vi "Tosca-Execute Flowchart.vi"(0 "Tosca":refnum<class "Parameters.lvclass">, 1 "StimCon":T1, 2 "IPC":T7, 7 "AODO":T4[](array[typedef]), 11 "error in":errorcluster, 13 "Control Refs":T9) -> (4 "Result":T8, 6 "History":string[](array[string]), 8 "Result string":string, 10 "Rxn time":i32, 14 "Abort":bool, 15 "error out":errorcluster)   [LabVIEW 2020]
uses:
  Typedefs/Tosca-Control Refs.ctl
  FSM Graph VIs/LV Source/FSM Editor/FSM Editor.xctl
  Typedefs/Tosca-Trial Result Enum.ctl
  IPC VIs/Tosca-IPC.ctl
  Classes/Parameters/Parameters.lvclass
  Digital Input VIs/Tosca-DI Queue Data.ctl
  Digital Input VIs/Tosca-Input Event.ctl
  Digital Input VIs/Tosca-Input Criterion.ctl
  epl-vi-lib/Utility VIs/Type Defs/Logic State.ctl
  Typedefs/Tosca-Accumulator.ctl
  Typedefs/Tosca-State AODO.ctl
  Typedefs/Tosca-AO Runtime.ctl
  Typedefs/Tosca-DO Runtime.ctl
  epl-vi-lib/Signal Synthesis VIs/4th Generation/Classes/SignalManager/SignalManager.lvclass
  Typedefs/Tosca-Synapse Start Data.ctl
  IPC VIs/Tosca-Message.ctl
  IPC VIs/Tosca-Message Action.ctl
  Typedefs/Tosca-Thread Type.ctl
  Imaging VIs/Tosca-2P-Notifier Data.ctl
  Typedefs/Tosca-MATLAB Queue Data.ctl
  Visual Stim VIs/Tosca-Grating.ctl
  Visual Stim VIs/Tosca-Grating Type.ctl
  Typedefs/Tosca-File IO Notification.ctl
  Typedefs/Tosca-SCL Element.ctl
  Typedefs/Tosca-Schedule Mode.ctl
  Typedefs/Tosca-Event Type.ctl
  Trace VIs/Tosca-Trace-Event.ctl
  Classes/Parameters/Parameters.lvclass/Parameters.ctl
  Classes/Parameters/Read Flowchart.vi
  Classes/Parameters/Read First state.vi
  Classes/Parameters/Read Target state.vi
  Classes/State/State.lvclass
panel:
  out "Tosca out":refnum<class "Parameters.lvclass">
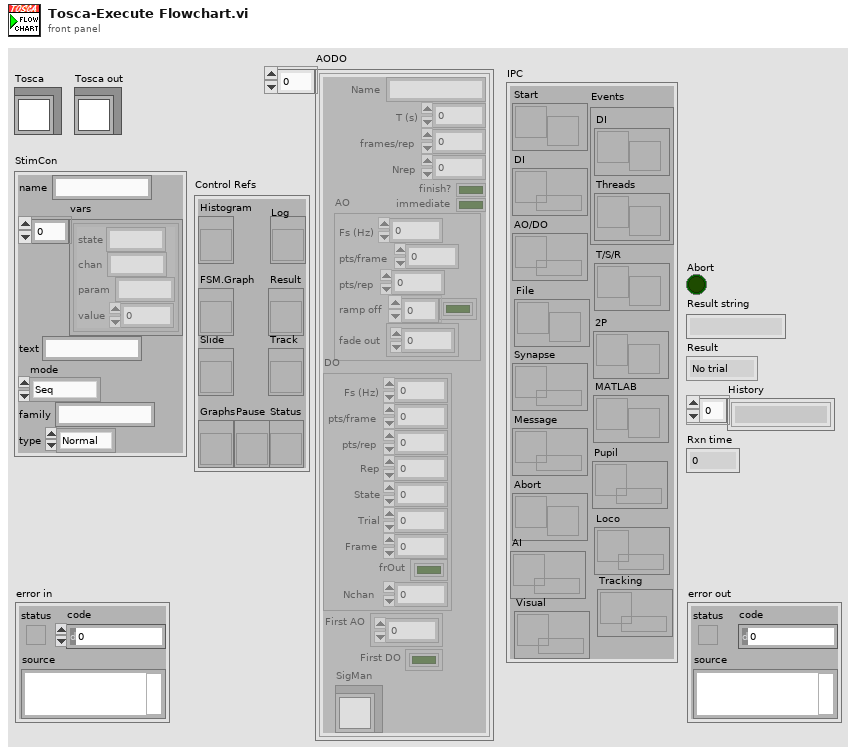
[diagram p1: front panel]
types:
  T1 = typedef "Tosca-SCL Element.ctl" = cluster{"name":string, "vars":cluster{"state":string, "chan":string, "param":string, "value":dbl}[], "text":string, "mode":T2, "family":string, "type":T3}
  T2 = typedef "Tosca-Schedule Mode.ctl" = enum16{"Seq", "CS+/CS-", "Adapt"}
  T3 = typedef "Tosca-Event Type.ctl" = enum16{"Normal", "CS+", "CS-"}
  T4 = typedef "Tosca-State AODO.ctl" = cluster{"Name":string, "T (s)":dbl, "First AO":dbl[][], "frames/rep":i32, "finish?":bool, "Nrep":i32, "AO":T5, "DO":T6, "immediate":bool, "First DO":bool[][], "SigMan":refnum<class "SignalManager.lvclass">}
  T5 = typedef "Tosca-AO Runtime.ctl" = cluster{"Fs (Hz)":dbl, "pts/frame":i32, "pts/rep":i32, "ramp off":bool[], "fade out":dbl[][]}
  T6 = typedef "Tosca-DO Runtime.ctl" = cluster{"Fs (Hz)":dbl, "pts/frame":i32, "pts/rep":i32, "Rep":i32, "State":i32, "Trial":i32, "Frame":i32, "frOut":bool[], "Nchan":i32}
  T7 = typedef "Tosca-IPC.ctl" = cluster{"Start":refnum<notifier>, "DI":refnum<queue>, "AO/DO":refnum<queue>, "Synapse":refnum<queue>, "Message":refnum<queue>, "Abort":refnum<notifier>, "Events":cluster{"DI":refnum<user-event>, "Threads ":refnum<user-event>}, "T/S/R":refnum<notifier>, "2P":refnum<notifier>, "MATLAB":refnum<notifier>, "Pupil":refnum<queue>, "Loco":refnum<queue>, "AI":refnum<queue>, "Tracking":refnum<queue>, "Visual":refnum<queue>, "File":refnum<notifier>}
  T8 = typedef "Tosca-Trial Result Enum.ctl" = enum16{"No trial", "Go", "No go", "Error", "Abort"}
  T9 = typedef "Tosca-Control Refs.ctl" = cluster{"FSM.Graph":refnum<vi>, "Slide":refnum<vi>, "Result":refnum<vi>, "Histogram":refnum<vi>, "Graphs":refnum<vi>, "Track":refnum<vi>, "Log":refnum<vi>, "Status":refnum<vi>, "Pause":refnum<vi>}
  T10 = typedef "Tosca-Trace-Event.ctl" = enum16{"Unspecified", "Trial start", "Enqueue", "Result", "End parser", "Frame", "Queue available", "Timeout sent", "WritePos", "TTL"}
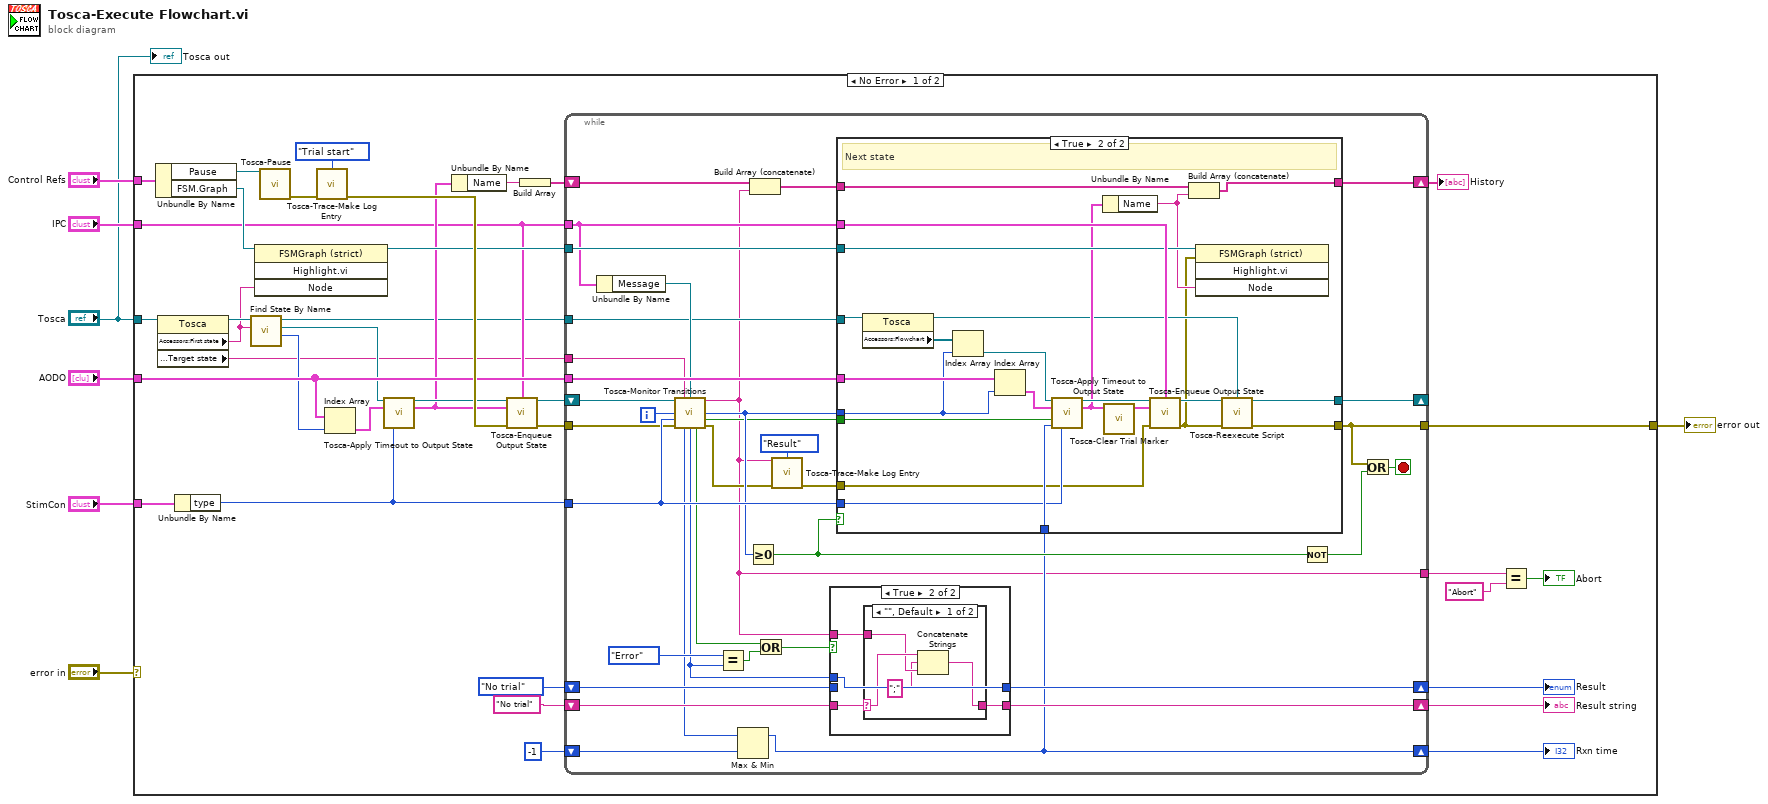
[diagram p0: block diagram]
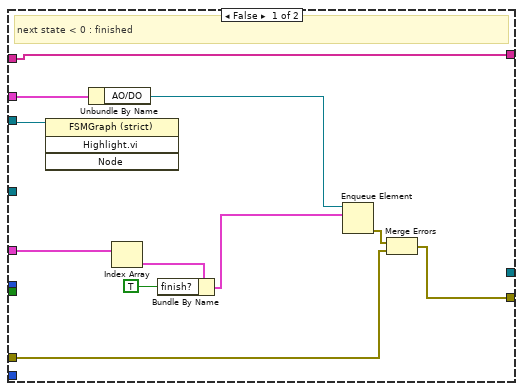
[diagram p4: hidden frame]
diagram:
  n1 = case shown="No Error" "error in" {
    selector: "error in" -> [_ w125]
    tunnel: "Control Refs" -> [w42 _]
    tunnel: "AODO" -> [w36 _]
    tunnel: [w31 w125] -> w5
    tunnel: "IPC" -> [w12 _]
    tunnel: "Tosca" -> [w22 _]
    tunnel: "StimCon" -> [w17 _]
    frame No Error {
      n2 = Unbundle By Name(w42) -> ("Pause"=w28:refnum<vi>, "FSM.Graph"=w24:refnum<vi>)
      n3 = property class="Tosca"(reference=w22) -> (reference out=w21:refnum<class "Parameters.lvclass">, "Accessors:First state"=w20:string, "Accessors:Target state"=w8:string)  [unwired: 1 in, 1 out]
      n4 = Unbundle By Name(w17) -> ("type"=w16:T3)
      n5 = call "Find State By Name.vi"("Name"=w20, "Tosca in"=w21) -> ("Index"=w19:i32, "State"=w15:refnum<class "State.lvclass">, "Tosca out"=w10:refnum<class "Parameters.lvclass">)  [unwired: 6 in, 1 out]
      n6 = invoke class="FSMGraph (strict)" method="Highlight.vi"(reference=w24, "Node"=w20) -> (reference out=w23:refnum<vi>)  [unwired: 2 in, 3 out]
      n7 = call "Tosca-Pause.vi"("Pause ref"=w28) -> ("error out"=w27:errorcluster)  [unwired: 14 in]
      n8 = call "Tosca-Trace-Make Log Entry.vi"("Event"=Tosca-Trace-Event."Trial start", "error in (no error)"=w27) -> ("error out"=w43:errorcluster)  [unwired: 13 in]
      n9 = Index Array(array=w36, index=w19) -> (element=w18:T4)
      n10 = call "Tosca-Apply Timeout to Output State.vi"("State"=w15, "AODO"=w18, "Trial type"=w16) -> ("State out"=w14:refnum<class "State.lvclass">, "AODO (out)"=w13:T4)  [unwired: 11 in]
      n11 = Unbundle By Name(w13) -> ("Name"=w40:string)
      n12 = call "Tosca-Enqueue Output State.vi"("State"=w14, "IPC"=w12, "AODO"=w13, "error in"=w43) -> ("State out"=w11:refnum<class "State.lvclass">, "error out"=w37:errorcluster)  [unwired: 10 in]
      n13 = Build Array(w40) -> (w39:string[])
      n14 = while {
        tunnel: w37 -> [w46]
        tunnel: w36 -> [w68]
        tunnel: w12 -> [w55]
        tunnel: [w70] -> w31
        tunnel: w23 -> [w76]
        tunnel: w16 -> [w75]
        shift-right: [w62] -> w35
        shift-left: Tosca-Trial_Result_Enum."No trial" ("Result") -> [w63]
        shift-right: [w72] -> w38
        shift-left: w39 -> [w74]
        tunnel: [w45] -> w9
        shift-right: [w60] -> w30
        shift-left: "No trial" -> [w61]
        shift-right: [w56] -> w25
        shift-left: -1 -> [w57]
        shift-right: [w51] -> _
        shift-left: w11 -> [w53]
        tunnel: w10 -> [w52]
        tunnel: w8 -> [w47]
        i -> [w66]
        stop <- w79 stop-if-true
        n15 = Unbundle By Name(w55) -> ("Message"=w54:refnum<queue>)
        n16 = call "Tosca-Monitor Transitions.vi"("Flow Element"=w53, "Decision state"=w47, "Message"=w54, "State"=w66, "Trial type"=w75, "error in"=w46) -> ("Result String"=w45:string, "Next"=w71:i32, "End on rep"=w69:bool, "Trxn"=w49:i32, "Result"=w48:T8, "named result"=w44:bool, "error out"=w64:errorcluster)  [unwired: 3 in]
        n17 = Equal?(x=Tosca-Trial_Result_Enum."Error" ("y"), y=w48) -> (x = y?=w50:bool)
        n18 = Max & Min(x=w49, y=w57) -> (max(x,y)=w56:i32)  [unwired: 1 out]
        n19 = Greater Or Equal To 0?(x=w71) -> (x >= 0?=w78:bool)
        n20 = Build Array (concatenate)(w74, w45) -> (w73:string[])
        n21 = Or(x=w44, y=w50) -> (x .or. y?=w58:bool)
        n22 = call "Tosca-Trace-Make Log Entry.vi"("Message"=w45, "Event"=Tosca-Trace-Event."Result", "error in (no error)"=w64) -> ("error out"=w65:errorcluster)  [unwired: 12 in]
        n23 = case shown="True" w58 {
          tunnel: w48 -> [_ w85]
          tunnel: w63 -> [w81 _]
          tunnel: [w81 w85] -> w62
          tunnel: w61 -> [w80 w84]
          tunnel: [w80 w82] -> w60
          tunnel: w45 -> [_ w83]
          frame False {
          }
          frame True {
            n24 = case shown="\"\", Default" w84 {
              selector: w84 -> [w89 _]
              tunnel: w83 -> [w88 w90]
              tunnel: [w87 w90] -> w82
              frame "", Default {
                n25 = Concatenate Strings(w89, ";", w88) -> (w87:string)
              }
              frame "No trial" {
              }
            }
          }
        }
        n26 = case shown="True" w78 {
          tunnel: w71 -> [_ w115]
          tunnel: w68 -> [w101 w124]
          tunnel: w55 -> [w98 w118]
          tunnel: w65 -> [w94 w109]
          tunnel: [w95 w104] -> w70
          tunnel: w76 -> [w91 w112]
          tunnel: w75 -> [_ w119]
          tunnel: w73 -> [w96 w123]
          tunnel: [w96 w122] -> w72
          tunnel: w69 -> [_ w110]
          tunnel: w56 -> [_ w120]
          tunnel: w52 -> [_ w117]
          tunnel: [_ w105] -> w51
          frame False {
            # "next state < 0 : finished"
            n27 = invoke class="FSMGraph (strict)" method="Highlight.vi"(reference=w91) -> ()  [unwired: 3 in, 4 out]
            n28 = Unbundle By Name(w98) -> ("AO/DO"=w92:refnum<queue>)
            n29 = Index Array(array=w101) -> (element=w100:T4)  [unwired: 1 in]
            n30 = Bundle By Name(cluster=w100, "finish?"=TRUE ("Continue?")) -> (w97:T4)
            n31 = Enqueue Element(queue=w92, element=w97) -> (error out=w99:errorcluster)  [unwired: 2 in, 2 out]
            n32 = Merge Errors(w99, w94) -> (w95:errorcluster)
          }
          frame True {
            # "Next state"
            n33 = property class="Tosca"(reference=w117) -> (reference out=w103:refnum<class "Parameters.lvclass">, "Accessors:Flowchart"=w116:refnum<class "State.lvclass">[])  [unwired: 1 in, 1 out]
            n34 = Index Array(array=w116, index=w115) -> (element=w114:refnum<class "State.lvclass">)
            n35 = Index Array(array=w124, index=w115) -> (element=w121:T4)
            n36 = call "Tosca-Apply Timeout to Output State.vi"("State"=w114, "AODO"=w121, "end on rep"=w110, "Trxn"=w120, "Trial type"=w119) -> ("State out"=w113:refnum<class "State.lvclass">, "AODO (out)"=w108:T4)  [unwired: 9 in]
            n37 = Unbundle By Name(w108) -> ("Name"=w111:string)
            n38 = call "Tosca-Clear Trial Marker.vi"("AODO"=w108) -> ("AODO Out"=w107:T4)  [unwired: 10 in]
            n39 = call "Tosca-Enqueue Output State.vi"("State"=w113, "IPC"=w118, "AODO"=w107, "error in"=w109) -> ("State out"=w106:refnum<class "State.lvclass">, "error out"=w102:errorcluster)  [unwired: 10 in]
            n40 = Build Array (concatenate)(w123, w111) -> (w122:string[])
            n41 = invoke class="FSMGraph (strict)" method="Highlight.vi"(reference=w112, error in=w102, "Node"=w111) -> ()  [unwired: 1 in, 4 out]
            n42 = call "Tosca-Reexecute Script.vi"("State in"=w106, "Tosca"=w103, "error in (no error)"=w102) -> ("State out"=w105:refnum<class "State.lvclass">, "error out"=w104:errorcluster)  [unwired: 11 in]
          }
        }
        n43 = Not(x=w78) -> (.not. x?=w77:bool)
        n44 = Or(x=w70, y=w77) -> (x .or. y?=w79:bool)
      }
      "Result" <- w35
      "History" <- w38
      "Result string" <- w30
      "Rxn time" <- w25
      n45 = Equal?(x=w9, y="Abort" ("x")) -> (x = y?=→"Abort":bool)
    }
    frame Error {
    }
  }
  "error out" <- w5
  "Tosca out" <- "Tosca"
